vi "Calibration on command(SubVI).vi"(10 "Calibrate":bool, 11 "File Path (Image Calibration 1)":path=path "\\\\hs2.lboro.ac.uk\\mmbc4/1_Univesity Work/Mechatronics/Machine Vision/Harry_Kane_Project/A3_table_cal_2.png") -> (0 "error out":errorcluster, 1 "Boolean":bool, 3 "Refnum out":T1(plugin-control))   [LabVIEW 2013]
uses:
  <vilib>/vision/driver/NI_Vision_Acquisition_Software.lvlib
panel:
  in  "Calibration image":path=path "\\\\hs2.lboro.ac.uk\\mmbc4/1_Univesity Work/Mechatronics/Machine Vision/Harry_Kane_Project/A3_table_cal_2.png"
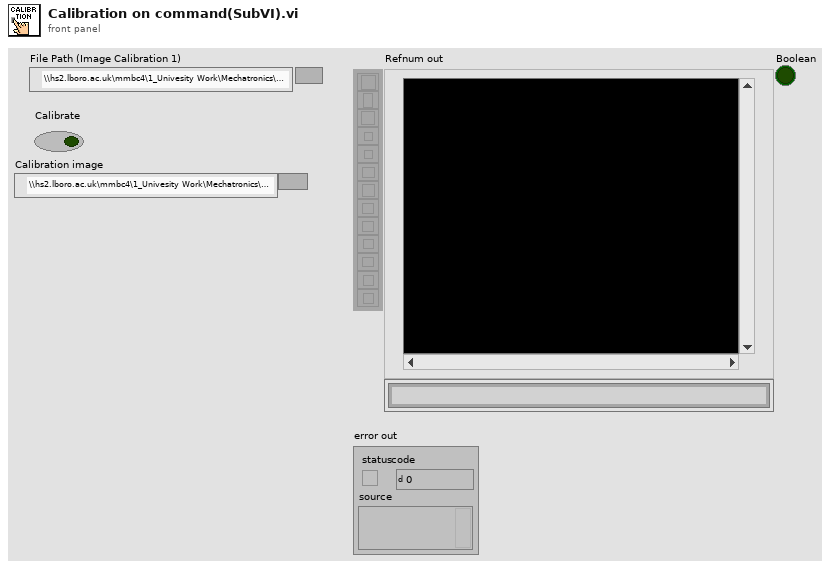
[diagram p1: front panel]
types:
  T1 = typedef "IMAQ Image.ctl" = refnum<image>
  T2 = typedef "Image Type" = u32
  T3 = typedef "IMAQdx.ctl" = refnum<k21>
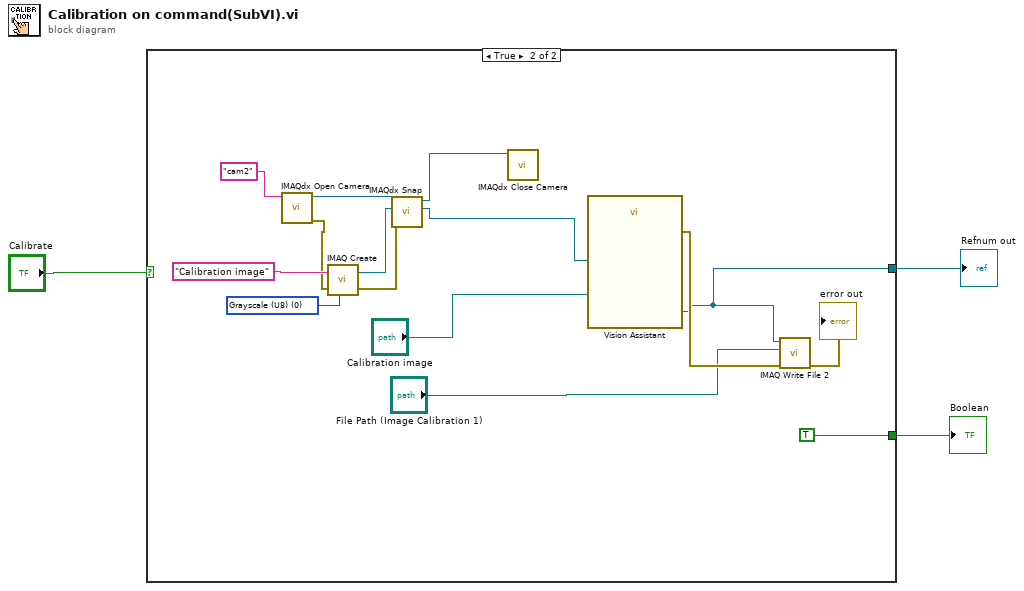
[diagram p0: block diagram]
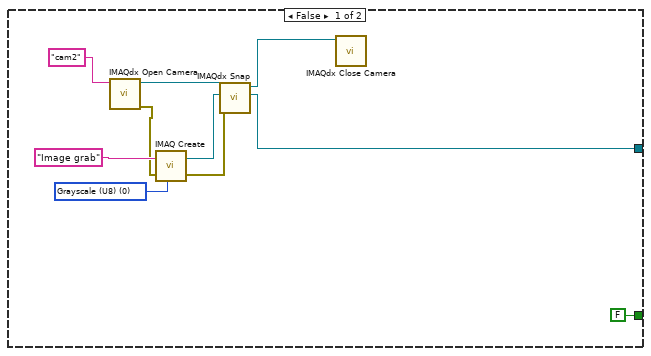
[diagram p2: hidden frame]
diagram:
  n1 = case shown="True" "Calibrate" {
    tunnel: [w5 w16] -> w3
    tunnel: [FALSE TRUE] -> w1
    frame False {
      w12 = T2 0 items=["Grayscale (U8)", "Grayscale (I16)", "Grayscale (SGL)", "Complex (CSG)", "RGB (U32)", "HSL (U32)", "RGB (U64)", "Grayscale (U16)"] ("Image Type")
      n2 = call <vilib>:"IMAQdx Open Camera.vi"("Session In"="cam2" ("Interface Name")) -> ("error out"=w6:errorcluster, "Session Out"=w7:T3)  [unwired: 9 in]
      n3 = call "IMAQ Create"("Image Name"="Image grab", "Image Type"=w12, "error in (no error)"=w6) -> ("New Image"=w11:T1, "error out"=w10:errorcluster)  [unwired: 2 in]
      n4 = call <vilib>:"IMAQdx Snap.vi"("error in"=w10, "Image In"=w11, "Session In"=w7) -> ("Image Out"=w5:T1, "Session Out"=w9:T3)  [unwired: 6 in, 1 out]
      n5 = call <vilib>:"IMAQdx Close Camera.vi"("Session In"=w9) -> ()  [unwired: 10 in, 1 out]
    }
    frame True {
      w27 = T2 0 items=["Grayscale (U8)", "Grayscale (I16)", "Grayscale (SGL)", "Complex (CSG)", "RGB (U32)", "HSL (U32)", "RGB (U64)", "Grayscale (U16)"] ("Image Type")
      n6 = call <vilib>:"IMAQdx Open Camera.vi"("Session In"="cam2" ("Interface Name")) -> ("error out"=w21:errorcluster, "Session Out"=w22:T3)  [unwired: 9 in]
      n7 = call "IMAQ Create"("Image Name"="Calibration image", "Image Type"=w27, "error in (no error)"=w21) -> ("New Image"=w26:T1, "error out"=w25:errorcluster)  [unwired: 2 in]
      n8 = call <vilib>:"IMAQdx Snap.vi"("error in"=w25, "Image In"=w26, "Session In"=w22) -> ("Image Out"=w20:T1, "Session Out"=w24:T3)  [unwired: 6 in, 1 out]
      n9 = call <vilib>:"IMAQdx Close Camera.vi"("Session In"=w24) -> ()  [unwired: 10 in, 1 out]
      n10 = call "Vision Assistant"("Image In"=w20, "File Path (Image Calibration 1)"="Calibration image") -> ("Image Out"=w16:T1, "error out"=w19:errorcluster)  [unwired: 24 in]
      n11 = call-poly "IMAQ Write File 2"("error in (no error)"=w19, "File Path"="File Path (Image Calibration 1)", "Image"=w16) -> ("error out"=→"error out":errorcluster)  [unwired: 7 in, 1 out]
    }
  }
  "Refnum out" <- w3
  "Boolean" <- w1
